vi "LXM32_Init.vi"(8 "error in":errorcluster, 11 "VISA resource name":refnum<visa-resource-name>) -> (0 "error out":errorcluster, 3 "VISA resource name out":refnum<visa-resource-name>)   [LabVIEW 2015, in "LXM32_Modbus_Serial.lvlib"]
uses:
  LXM32_Modbus_Serial.lvlib
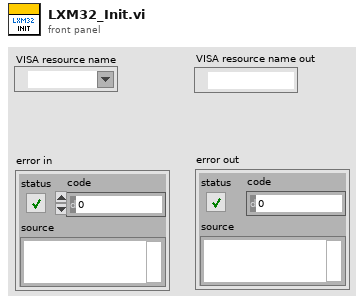
[diagram p1: front panel]
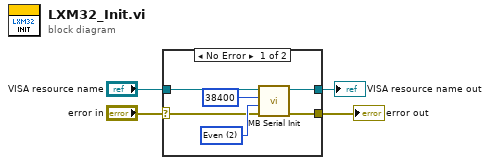
[diagram p0: block diagram]
diagram:
  n1 = case shown="No Error" "error in" {
    selector: "error in" -> [w7 w11]
    tunnel: "VISA resource name" -> [w8 _]
    tunnel: [w6 _] -> w1
    tunnel: [w5 w11] -> w2
    frame No Error {
      w10 = u16 2 items=["None", "Odd", "Even", "Mark", "Space"] ("Parity")
      n2 = call "MB Serial Init.vi"("error in (no error)"=w7, "Parity"=w10, "Baud Rate"=u32 38400, "VISA resource name"=w8) -> ("error out"=w5:errorcluster, "VISA resource name out"=w6:refnum<visa-resource-name>)  [unwired: 6 in]
    }
    frame Error {
    }
  }
  "error out" <- w2
  "VISA resource name out" <- w1
